vi "5_31_Fxp_addation.vi"(1 "y":fxp<+/-,31,5>, 2 "x":fxp<+/-,31,5>) -> (0 "x+y":fxp<+/-,32,6> format="%.41g")   [LabVIEW 2020]
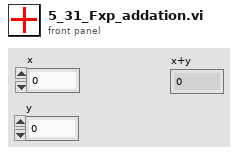
[diagram p1: front panel]
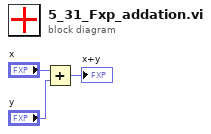
[diagram p0: block diagram]
diagram:
  n1 = Add(x="x", y="y") -> (x+y=→"x+y":fxp<+/-,32,6>)
